vi "showProgressBarServer(SubVI).vi"(10 "file size":i64, 11 "to be transmitted":i64) -> (3 "progress bar":dbl(slide) scale=0.0..100.0)   [LabVIEW 2021]
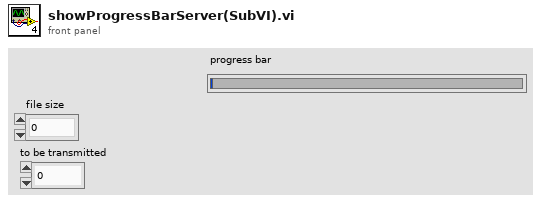
[diagram p1: front panel]
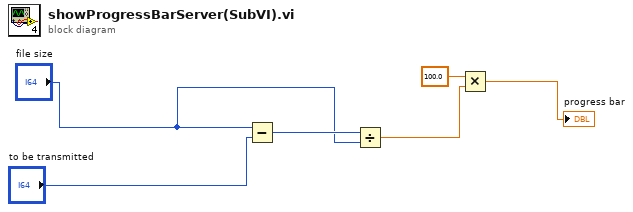
[diagram p0: block diagram]
diagram:
  n1 = Subtract(x="file size", y="to be transmitted") -> (x-y=w5:i64)
  n2 = Divide(x=w5, y="file size") -> (x/y=w3:dbl)
  n3 = Multiply(x=100.0, y=w3) -> (x*y=→"progress bar":dbl)
